vi "FITS line pad length.vi"(8 "error in (no error)":errorcluster, 11 "Line":string) -> (0 "error out":errorcluster, 3 "Padded Line":string)   [LabVIEW 2020]
panel:
  out "length":i32
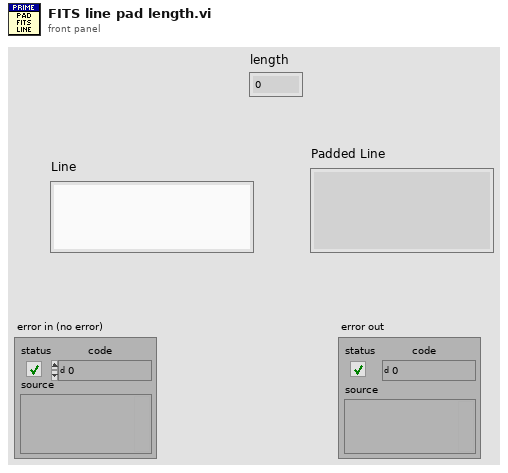
[diagram p1: front panel]
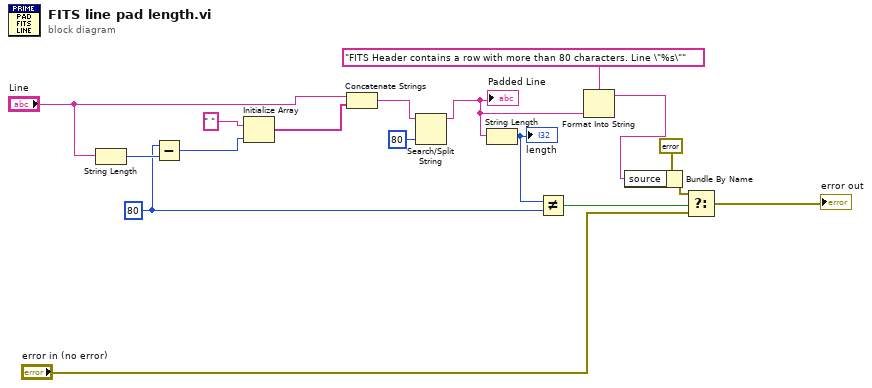
[diagram p0: block diagram]
diagram:
  w5 = 80
  n1 = String Length(string="Line") -> (length=w6:i32)
  n2 = Subtract(x=w5, y=w6) -> (x-y=w4:i32)
  n3 = Initialize Array(" ", w4) -> (w15:string[])
  n4 = Concatenate Strings("Line", w15) -> (w2:string)
  n5 = Search/Split String(string=w2, offset (0)=80) -> (substring before match=w1:string)  [unwired: 1 in, 2 out]
  "Padded Line" <- w1
  n6 = String Length(string=w1) -> (length=w14:i32)
  "length" <- w14
  n7 = Not Equal?(x=w14, y=w5) -> (x != y?=w13:bool)
  n8 = Format Into String(format string="FITS Header contains a row with more than 80 characters. Line \"%s\"" ("source"), w1) -> (resulting string=w8:string)  [unwired: 2 in, 1 out]
  n9 = Bundle By Name(cluster=errorcluster {"status"=TRUE, "code"=5000, "source"="FITS Header contains a row with more than 80 characters."} ("s? t:f"), "source"=w8) -> (w7:errorcluster)
  n10 = Select(t=w7, s=w13, f="error in (no error)") -> (s? t:f=→"error out":errorcluster)
